vi "c ctre phoenixpro Request Control BMS Manual Vboost.vi"(0 "canbus":string, 1 "cancelOtherRequests":bool, 5 "ecuEncoding":u32, 9 "updateTime":dbl, 11 "error in (no error)":errorcluster, 12 "EnableClosedLoop":bool, 13 "TargetVoltage":dbl, 14 "TargetDutyCycle":dbl) -> (4 "function return":i32, 15 "error out":errorcluster)   [LabVIEW 2020, in "CTRE_PhoenixTools.lvlib"]
doc: "CTREXPORT int c_ctre_phoenixpro_RequestControlBMSManualVboost(const char *canbus, uint32_t ecuEncoding, double updateTime, bool cancelOtherRequests, bool EnableClosedLoop, double TargetVoltage, double TargetDutyCycle);"
uses:
  <userlib>/CTRE_PhoenixTools/CTRE_PhoenixTools.lvlib
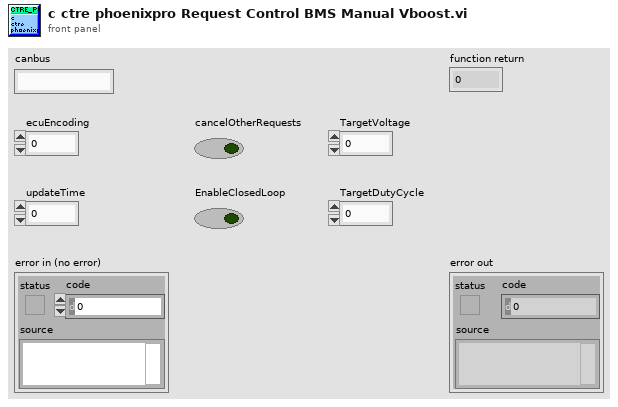
[diagram p1: front panel]
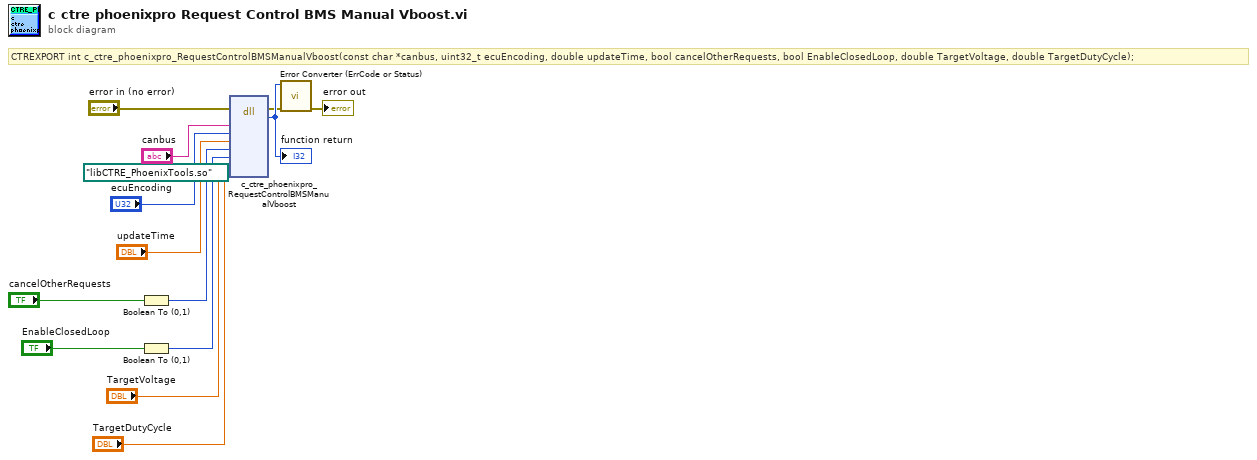
[diagram p0: block diagram]
diagram:
  # "CTREXPORT int c_ctre_phoenixpro_RequestControlBMSManualVboost(const char *canbus, uint32_t ecuEncoding, double updateTime, bool cancelOtherRequests, bool EnableClosedLoop, double TargetVoltage, double TargetDutyCycle);"
  n1 = Boolean To (0,1)(Boolean="cancelOtherRequests") -> (0, 1=w9:i16)
  n2 = Boolean To (0,1)(Boolean="EnableClosedLoop") -> (0, 1=w7:i16)
  n3 = dll-call lib="?" fn="c_ctre_phoenixpro_RequestControlBMSManualVboost"(path in=path "libCTRE_PhoenixTools.so", error in="error in (no error)", "canbus"="canbus", "ecuEncoding"="ecuEncoding", "updateTime"="updateTime", "cancelOtherRequests"=w9, "EnableClosedLoop"=w7, "TargetVoltage"="TargetVoltage", "TargetDutyCycle"="TargetDutyCycle") -> (error out=w3:errorcluster, "return type"=w14:i32)  [unwired: 8 in, 1 out]
  "function return" <- w14
  n4 = call <userlib>:"Error Converter (ErrCode or Status).vi"("error in (no error)"=w3, "error code"=w14) -> ("error out"=→"error out":errorcluster)  [unwired: 9 in]
